vi "Read Key (Path).vi"(7 "section":string, 8 "error in (no error)":errorcluster, 9 "default value":path, 10 "key":string, 11 "refnum":T1) -> (0 "error out":errorcluster, 1 "value":path, 2 "found?":bool, 3 "refnum out":T1)   [LabVIEW 2020, in "NI_LVConfig.lvlib"]
doc: "Reads a value associated with a key in a specified section from the configuration data identified by <B>refnum</B>. If the key does not exist, the VI returns the default value. This VI supports multibyte characters in strings. Wire data to the <B>default value</B> input to determine the polymorphic instance to use or manually select the instance."
uses:
  NI_LVConfig.lvlib
  Config Data RefNum.ctl
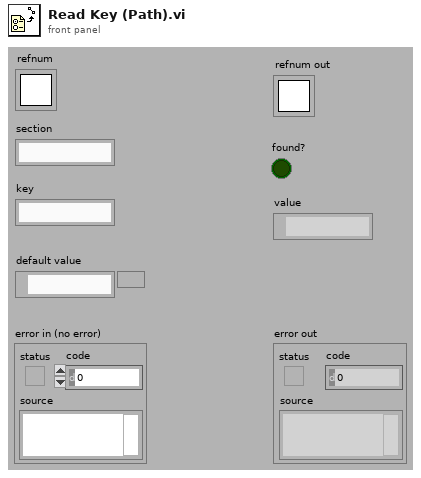
[diagram p1: front panel]
types:
  T1 = typedef "NI_LVConfig.lvlib/Config Data RefNum.ctl" = refnum<k1>
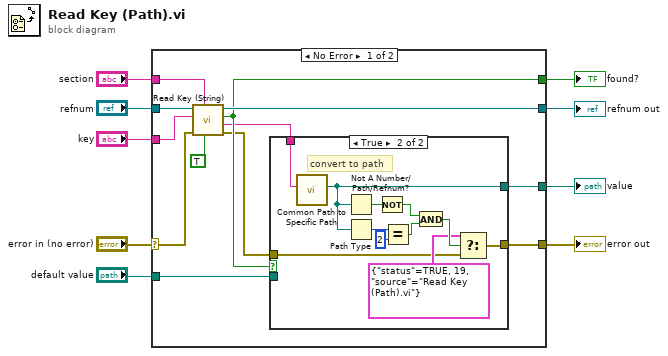
[diagram p0: block diagram]
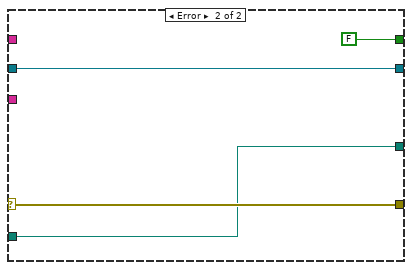
[diagram p3: hidden frame]
diagram:
  n1 = case shown="No Error" "error in (no error)" {
    selector: "error in (no error)" -> [w14 w38]
    tunnel: [w21 w38] -> w8
    tunnel: "section" -> [w18 _]
    tunnel: "key" -> [w12 _]
    tunnel: "default value" -> [w19 w37]
    tunnel: [w15 FALSE ("key exists?")] -> w5
    tunnel: [w20 w37] -> w3
    tunnel: "refnum" -> [w17 w35]
    tunnel: [w16 w35] -> w1
    frame No Error {
      n2 = call "Read Key (String).vi"("read raw string? (F)"=TRUE, "section"=w18, "error in (no error)"=w14, "key"=w12, "refnum"=w17) -> ("error out"=w13:errorcluster, "value"=w11:string, "found?"=w15:bool, "refnum out"=w16:T1)  [unwired: 3 in]
      n3 = case shown="True" w15 {
        tunnel: w11 -> [_ w24]
        tunnel: w19 -> [w23 _]
        tunnel: [w23 w25] -> w20
        tunnel: w13 -> [w22 w26]
        tunnel: [w22 w28] -> w21
        frame False {
        }
        frame True {
          # "convert to path"
          n4 = call "Common Path to Specific Path.vi"("common path"=w24) -> ("specific path"=w25:path)  [unwired: 10 in]
          n5 = Not A Number/Path/Refnum?(number/path/refnum=w25) -> (NaN/Path/Refnum?=w32:bool)
          n6 = Path Type(1:w25) -> (0:w34:i16)
          n7 = Not(x=w32) -> (.not. x?=w31:bool)
          n8 = Equal?(x=w34, y=i16 2) -> (x = y?=w30:bool)
          n9 = And(x=w31, y=w30) -> (x .and. y?=w29:bool)
          n10 = Select(t=cluster{"status":bool, u16, "source":string} {"status"=TRUE, 19, "source"="Read Key (Path).vi"} ("f"), s=w29, f=w26) -> (s? t:f=w28:errorcluster)
        }
      }
    }
    frame Error {
    }
  }
  "error out" <- w8
  "found?" <- w5
  "value" <- w3
  "refnum out" <- w1
